vi "getPacketType.vi"(10 "Packet First Byte":u8 format="%08b") -> (2 "Control Packet Type":T1)   [LabVIEW 2013, in "ControlPacket.lvclass"]
uses:
  ControlPacket.lvclass
  Control Packet Type -- enum.ctl
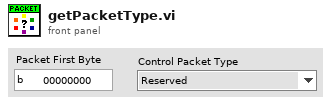
[diagram p1: front panel]
types:
  T1 = typedef "ControlPacket.lvclass/Control Packet Type -- enum.ctl" = enum16{"Reserved", "CONNECT", "CONNACK", "PUBLISH", "PUBACK", "PUBREC", "PUBREL", "PUBCOMP", "SUBSCRIBE", "SUBACK", "UNSUBSCRIBE", "UNSUBACK", "PINGREQ", "PINGRESP", "DISCONNECT", "Reserved(15)"}
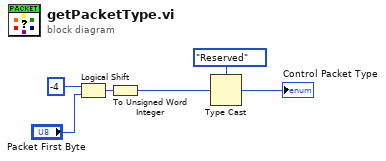
[diagram p0: block diagram]
diagram:
  n1 = Logical Shift(y=i16 -4, x="Packet First Byte") -> (x << y=w3:u8)
  n2 = To Unsigned Word Integer(number=w3) -> (unsigned 16bit integer=w4:u16)
  n3 = Type Cast(type=Control_Packet_Type_--_enum."Reserved" ("Control Packet Type"), x=w4) -> (*(type *) &x=→"Control Packet Type":T1)
